vi "Encoder rotations to feet.vi"(10 "Encoder Rotations":dbl) -> (2 "Feet":dbl)   [LabVIEW 2017]
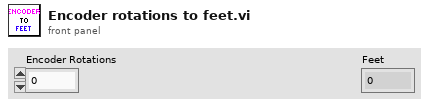
[diagram p1: front panel]
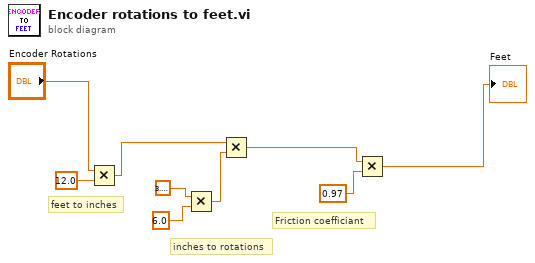
[diagram p0: block diagram]
diagram:
  # "inches to rotations"
  # "feet to inches"
  # "Friction coefficiant"
  n1 = Multiply(x="Encoder Rotations", y=12.0) -> (x*y=w5:dbl)
  n2 = Multiply(x=3.141592653589793, y=6.0) -> (x*y=w4:dbl)
  n3 = Multiply(x=w5, y=w4) -> (x*y=w1:dbl)
  n4 = Multiply(x=w1, y=0.97) -> (x*y=→"Feet":dbl)
